vi "New Configuration to Session.vi"(8 "error in":errorcluster, 11 "config data ref in":T1) -> (0 "error out":errorcluster, 3 "config data ref out":T1)   [LabVIEW 2017, in "DSF Core.lvlib" / "Configuration Session.lvclass"]
uses:
  Configuration Session.lvclass
  DSF Config Data Ref.ctl
  DSF Config Data.ctl
  Internal DSF Configuration.ctl
  Typedefs/DSF Version Info.ctl
  Internal DSF Plugin with ID.ctl
  Internal DSF Plugin Info.ctl
  Typedefs/DSF Timing Info.ctl
  Typedefs/DSF Engine Plugin Thread Configuration.ctl
  Typedefs/DSF Settings Info.ctl
  Internal DSF Group with ID.ctl
  Internal DSF Group Info.ctl
  Internal DSF Transfer with ID.ctl
  Internal DSF Transfer Info.ctl
  Internal DSF Channel with ID.ctl
  Internal DSF Channel Info.ctl
  Internal DSF Settings with ID.ctl
  Internal DSF Settings Info.ctl
  DSF Core.lvlib
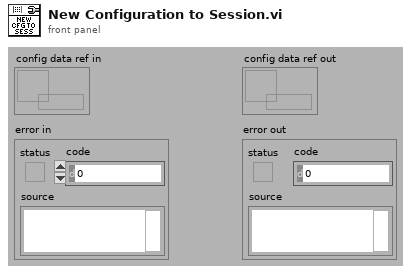
[diagram p1: front panel]
types:
  T1 = typedef "DSF Core.lvlib/Configuration Session.lvclass/DSF Config Data Ref.ctl" = refnum<data-value>
  T2 = typedef "DSF Core.lvlib/DSF Version Info.ctl" = cluster{"major":u32, "minor":u32, "fix":u32, "build":string}
  T3 = typedef "DSF Core.lvlib/Configuration Session.lvclass/Internal DSF Configuration.ctl" = cluster{"dsfversion":T2, "version":T2, "plugins":T4[], "groups":T9[], "transfers":T11[], "channels":T13[], "settings":T15[]}
  T4 = typedef "DSF Core.lvlib/Configuration Session.lvclass/Internal DSF Plugin with ID.ctl" = cluster{"id":string, "values":T5}
  T5 = typedef "DSF Core.lvlib/Configuration Session.lvclass/Internal DSF Plugin Info.ctl" = cluster{"components":string[], "timing":T6, "group ids":string[], "settings id":string, "threads":T7[]}
  T6 = typedef "DSF Core.lvlib/DSF Timing Info.ctl" = cluster{"priority":u64, "decimation":u64, "offset":u64}
  T7 = typedef "DSF Core.lvlib/DSF Engine Plugin Thread Configuration.ctl" = cluster{"buffer converter settings":T8, "transceiver settings":T8, "processor":i32, "priority offset":i16}
  T8 = typedef "DSF Core.lvlib/DSF Settings Info.ctl" = cluster{"key":string, "value":string}[]
  T9 = typedef "DSF Core.lvlib/Configuration Session.lvclass/Internal DSF Group with ID.ctl" = cluster{"id":string, "values":T10}
  T10 = typedef "DSF Core.lvlib/Configuration Session.lvclass/Internal DSF Group Info.ctl" = cluster{"direction":i32, "timing":T6, "transfer ids":string[], "settings id":string, "thread":i32, "timeout behavior":u8}
  T11 = typedef "DSF Core.lvlib/Configuration Session.lvclass/Internal DSF Transfer with ID.ctl" = cluster{"id":string, "values":T12}
  T12 = typedef "DSF Core.lvlib/Configuration Session.lvclass/Internal DSF Transfer Info.ctl" = cluster{"byte order":i32, "channel ids":string[], "settings id":string}
  T13 = typedef "DSF Core.lvlib/Configuration Session.lvclass/Internal DSF Channel with ID.ctl" = cluster{"id":string, "values":T14}
  T14 = typedef "DSF Core.lvlib/Configuration Session.lvclass/Internal DSF Channel Info.ctl" = cluster{"string buffer offset":u64, "string data type":i32, "engine data type":i32, "settings id":string}
  T15 = typedef "DSF Core.lvlib/Configuration Session.lvclass/Internal DSF Settings with ID.ctl" = cluster{"id":string, "values":T16}
  T16 = typedef "DSF Core.lvlib/Configuration Session.lvclass/Internal DSF Settings Info.ctl" = cluster{"key":string, "value":string}[]
  T17 = typedef "DSF Core.lvlib/Configuration Session.lvclass/DSF Config Data.ctl" = cluster{"dsf configuration":T3, "path":path, "dirty":bool}
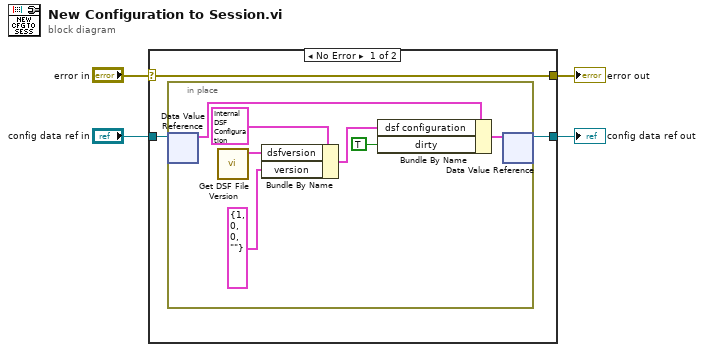
[diagram p0: block diagram]
diagram:
  n1 = case shown="No Error" "error in" {
    selector: "error in" -> [w7 w15]
    tunnel: [w7 w15] -> w4
    tunnel: [w5 w16] -> w1
    tunnel: "config data ref in" -> [w6 w16]
    frame No Error {
      n2 = in-place {
        n3 = in-place-dvr #1(w6) -> (w8:T17)  [unwired: 1 out]
        n4 = call "Get DSF File Version.vi"() -> ("dsf"=w11:T2)  [unwired: 11 in]
        n5 = Bundle By Name(cluster=T3 {"dsfversion"={"major"=0, "minor"=0, "fix"=0, "build"=""}, "version"={"major"=0, "minor"=0, "fix"=0, "build"=""}, "plugins"=[], "groups"=[], "transfers"=[], "channels"=[], "settings"=[]} ("dsf configuration"), "dsfversion"=w11, "version"=T2 {"major"=1, "minor"=0, "fix"=0, "build"=""}) -> (w12:T3)
        n6 = Bundle By Name(cluster=w8, "dsf configuration"=w12, "dirty"=TRUE) -> (w9:T17)
        n7 = in-place-dvr #1(w9) -> (w5:T1)  [unwired: 1 out]
      }
    }
    frame Error {
    }
  }
  "error out" <- w4
  "config data ref out" <- w1
